vi "subvi_window_test.vi"() -> ()   [LabVIEW 2018]
panel:
  in  "Title_Str":string
  in  "Close_Btn":bool
  in  "Output_Btn":bool
  in  "Mark_Btn":bool=TRUE
  in  "Info_Listbox":i32(listbox)=-1
  in  "Mass_Graph":cluster{"X":dbl[], "Y":dbl[]}[](graph)=[{"X"=[0.0], "Y"=[0.0]}, {"X"=[0.0], "Y"=[0.0]}]
  out "Ctrl Ref":refnum<vi>[](array[refnum])
  in  "Enum":enum16{"zoom in", "Select Range"}(ring)
  out "Ctrl Name":string[](array[string])
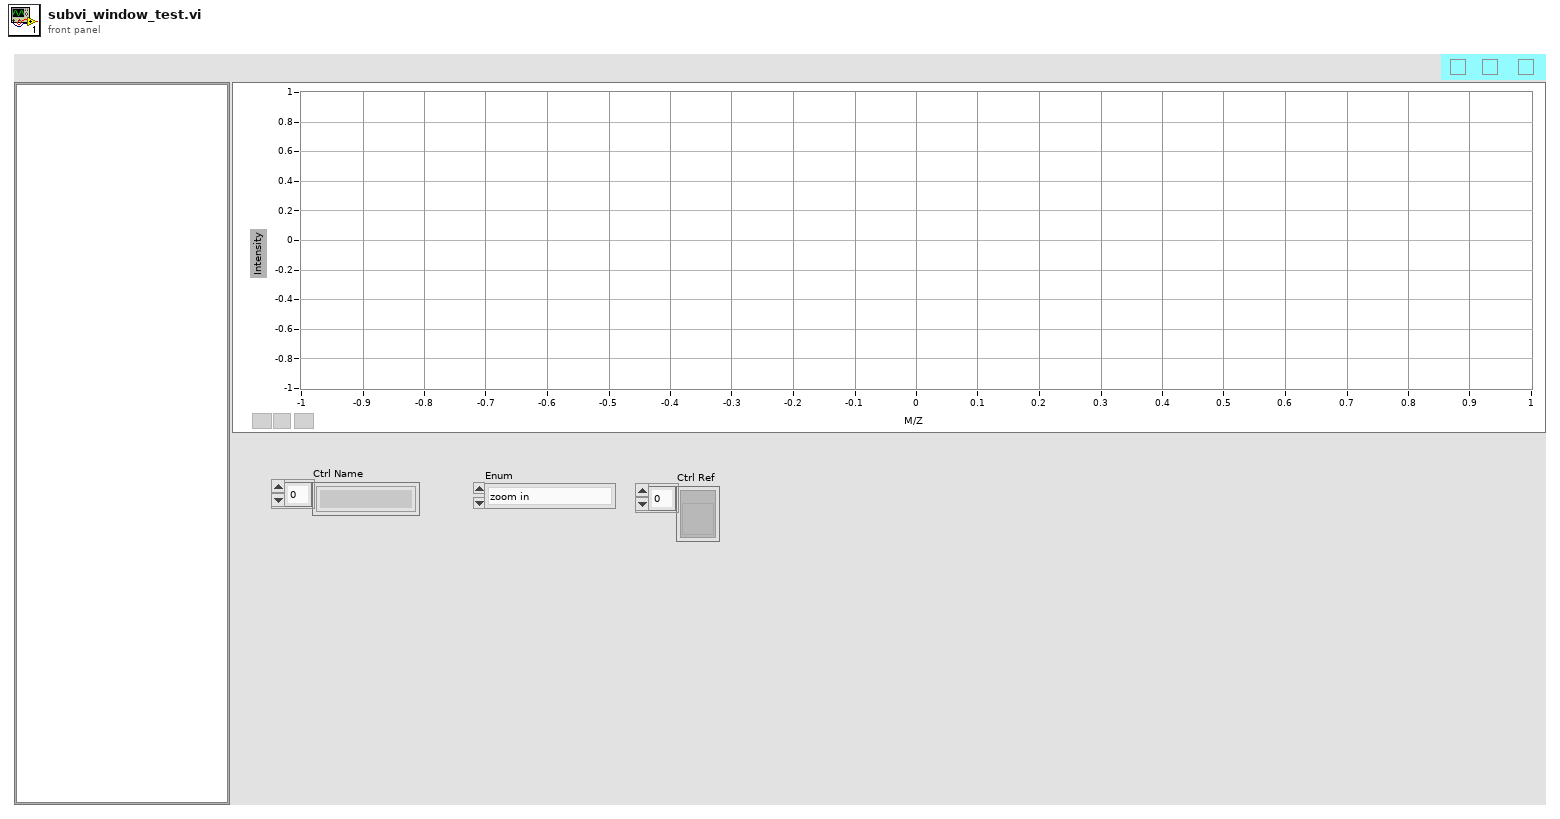
[diagram p1: front panel]
types:
  T1 = cluster{"Title_Str":refnum<vi>, "Mass_Graph":refnum<vi>, "Enum":refnum<vi>, "Info_Listbox":refnum<vi>, "Ctrl Ref":refnum<vi>, "Ctrl Name":refnum<vi>, "Mark_Btn":refnum<vi>, "Output_Btn":refnum<vi>, "Close_Btn":refnum<vi>}
  T2 = enum8{"Enabled", "Disabled", "Disabled and Grayed Out"}
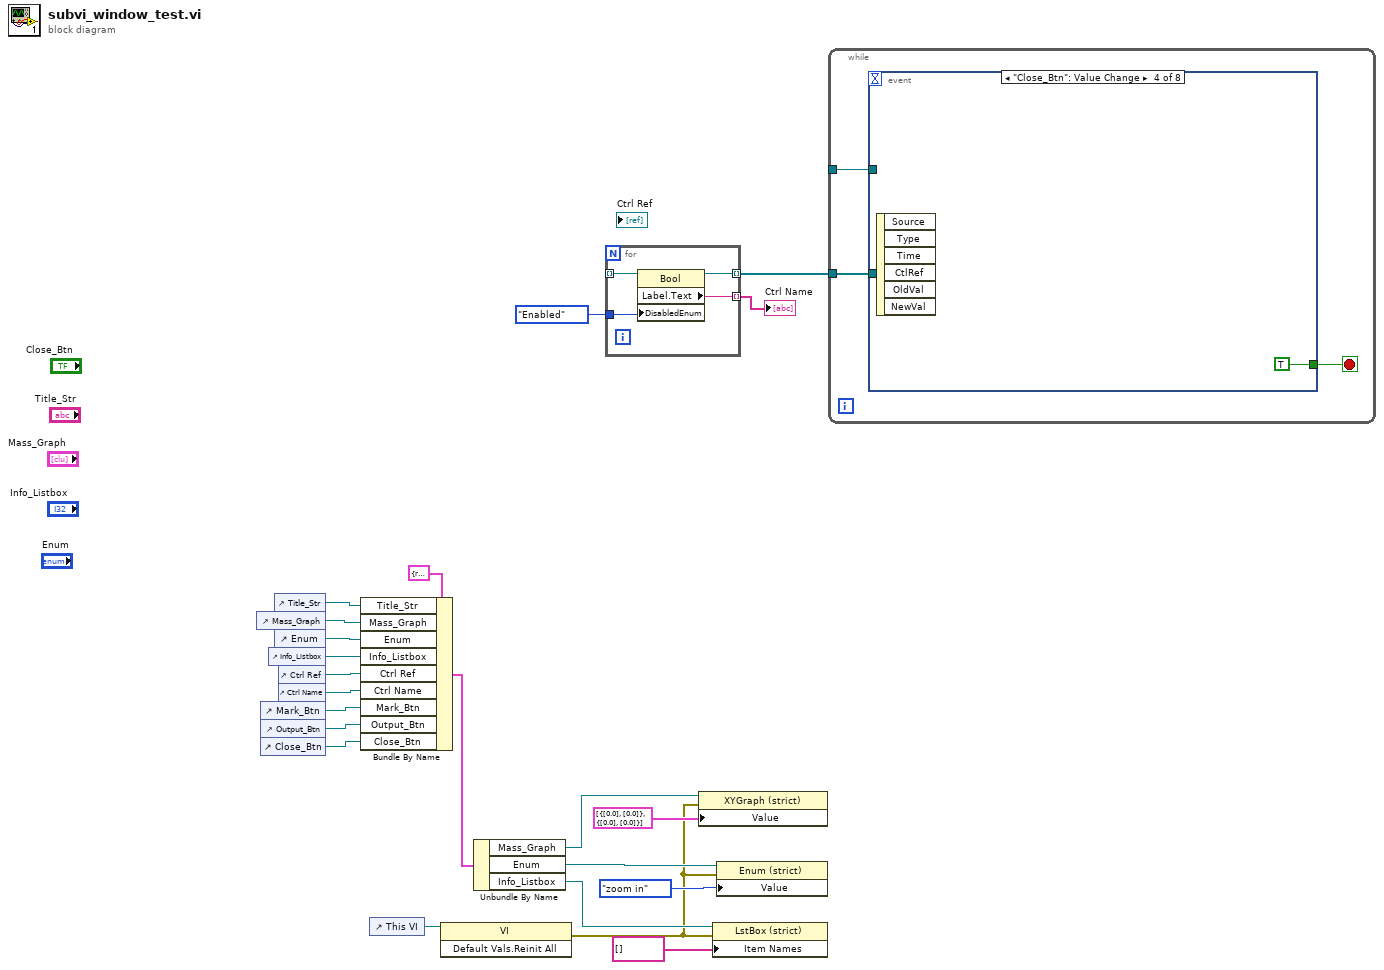
[diagram p0: block diagram]
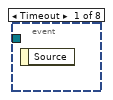
[diagram p2: hidden frame]
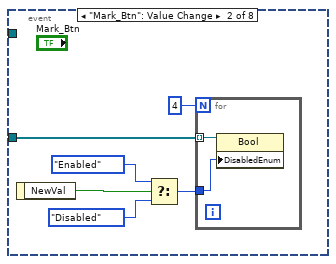
[diagram p3: hidden frame]
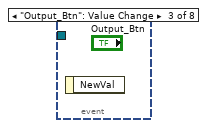
[diagram p4: hidden frame]
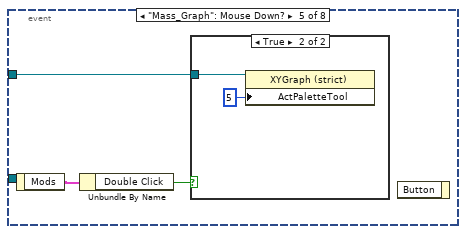
[diagram p5: hidden frame]
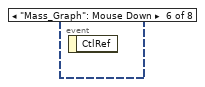
[diagram p7: hidden frame]
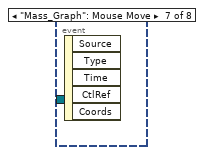
[diagram p8: hidden frame]
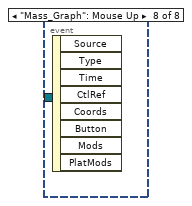
[diagram p9: hidden frame]
diagram:
  n1 = control-ref of="Mass_Graph"() -> (w14:refnum<vi>)
  n2 = control-ref of="Mark_Btn"() -> (w9:refnum<vi>)
  n3 = control-ref of="Output_Btn"() -> (w8:refnum<vi>)
  n4 = control-ref of="Close_Btn"() -> (w7:refnum<vi>)
  n5 = control-ref of="Info_Listbox"() -> (w12:refnum<vi>)
  n6 = control-ref of="Title_Str"() -> (w15:refnum<vi>)
  n7 = control-ref of="Enum"() -> (w13:refnum<vi>)
  n8 = control-ref of="Ctrl Ref"() -> (w11:refnum<vi>)
  n9 = control-ref of="Ctrl Name"() -> (w10:refnum<vi>)
  n10 = Bundle By Name(cluster=T1 {"Title_Str"=refnum, "Mass_Graph"=refnum, "Enum"=refnum, "Info_Listbox"=refnum, "Ctrl Ref"=refnum, "Ctrl Name"=refnum, "Mark_Btn"=refnum, "Output_Btn"=refnum, "Close_Btn"=refnum}, "Title_Str"=w15, "Mass_Graph"=w14, "Enum"=w13, "Info_Listbox"=w12, "Ctrl Ref"=w11, "Ctrl Name"=w10, "Mark_Btn"=w9, "Output_Btn"=w8, "Close_Btn"=w7) -> (w6:T1)
  n11 = control-ref of="This VI"() -> (w19:refnum<vi>)
  n12 = invoke class="VI" method="Default Vals.Reinit All"(reference=w19) -> (error out=w1:errorcluster)  [unwired: 2 in, 2 out]
  n13 = Unbundle By Name(w6) -> ("Mass_Graph"=w5:refnum<vi>, "Enum"=w4:refnum<vi>, "Info_Listbox"=w2:refnum<vi>)
  n14 = for {
    tunnel: _ -> [w26] mode=indexing
    tunnel: [w25] -> w17 mode=indexing
    tunnel: [w24] -> w18 mode=indexing
    tunnel: T2."Enabled" ("Disabled") -> [w23]
    n15 = property class="Bool"(reference=w26, "DisabledEnum"=w23) -> (reference out=w24:refnum<vi>, "Label.Text"=w25:string)  [unwired: 1 in, 1 out]
  }
  "Ctrl Name" <- w17
  n16 = property class="XYGraph (strict)"(reference=w5, error in=w1, "Value"=cluster{"X":dbl[], "Y":dbl[]}[] [{"X"=[0.0], "Y"=[0.0]}, {"X"=[0.0], "Y"=[0.0]}]) -> ()  [unwired: 2 out]
  n17 = property class="LstBox (strict)"(reference=w2, error in=w1, "Item Names"=string[] []) -> ()  [unwired: 2 out]
  n18 = property class="Enum (strict)"(reference=w4, error in=w1, "Value"=enum16{"zoom in", "Select Range"}."zoom in") -> ()  [unwired: 2 out]
  n19 = while {
    tunnel: w18 -> [w29]
    tunnel: _ -> [w28]
    stop <- w27 stop-if-true
    n20 = event shown="[3] \"Close_Btn\": Value Change" {
      selector: _ -> [_ _ _ _ _ _ _ _]
      dyn-events: _ -> [_ _ _ _ _ _ _ _]
      timeout: _ -> [_ _ _ _ _ _ _ _]
      tunnel: w29 -> [_ w33 _ _ _ _ _ _]
      tunnel: w28 -> [_ _ _ _ w39 _ _ _]
      tunnel: [_ _ _ TRUE _ _ _ _] -> w27
      event Timeout {
        n21 = event-data() -> ()  [unwired: 1 in, 1 out]
      }
      event "Mark_Btn": Value Change {
        n22 = event-data() -> ("NewVal"=w35:bool)  [unwired: 1 in]
        n23 = Select(t=T2."Enabled" ("Disabled"), s=w35, f=T2."Disabled") -> (s? t:f=w30:T2)
        n24 = for {
          N: 4 -> [_]
          tunnel: w33 -> [w37] mode=indexing
          tunnel: w30 -> [w36]
          n25 = property class="Bool"(reference=w37, "DisabledEnum"=w36) -> ()  [unwired: 1 in, 2 out]
        }
      }
      event "Output_Btn": Value Change {
        n26 = event-data() -> ()  [unwired: 1 in, 1 out]
      }
      event "Close_Btn": Value Change {
        n27 = event-data() -> ()  [unwired: 1 in, 6 out]
      }
      event "Mass_Graph": Mouse Down? {
        n28 = event-data() -> ("Mods"=w41:cluster{"Double Click":bool, "Menu Key":bool})  [unwired: 1 in]
        n29 = Unbundle By Name(w41) -> ("Double Click"=w40:bool)
        n30 = case shown="True" w40 {
          tunnel: w39 -> [_ w43]
          frame False {
          }
          frame True {
            n31 = property class="XYGraph (strict)"(reference=w43, "ActPaletteTool"=5 ("Palette:Active Tool")) -> ()  [unwired: 1 in, 2 out]
          }
        }
        n32 = event-data() -> ()  [unwired: 2 in, 1 out]
      }
      event "Mass_Graph": Mouse Down {
        n33 = event-data() -> ()  [unwired: 1 in, 1 out]
      }
      event "Mass_Graph": Mouse Move {
        n34 = event-data() -> ()  [unwired: 1 in, 5 out]
      }
      event "Mass_Graph": Mouse Up {
        n35 = event-data() -> ()  [unwired: 1 in, 8 out]
      }
    }
  }
